vi "Fit Hall.vi"(11 "File Path":path=path "\\\\myhome\\NHMFL/Projects/Pressure/Code/Alex/m005_092123.tdms") -> ()   [LabVIEW 2023]
uses:
  <vilib>/Utility/file.llb/Write Delimited Spreadsheet (DBL).vi
  <vilib>/Analysis/NI_AALPro.lvlib
panel:
  in  "Save?":bool
  out "Waveform Graph":dbl[](graph)
  in  "X (Temperature)":dbl
  in  "file path (Fit results)":path
  out "Polynomial Coefficients":dbl[](array[numeric])
  in  "polynomial order":i32=2
  in  "Y":string="LakeShore 370 (18) R"
  in  "X":string="B"
  out "XY Graph":cluster{dbl[], dbl[]}[](graph)
  in  "group name in":string="p"
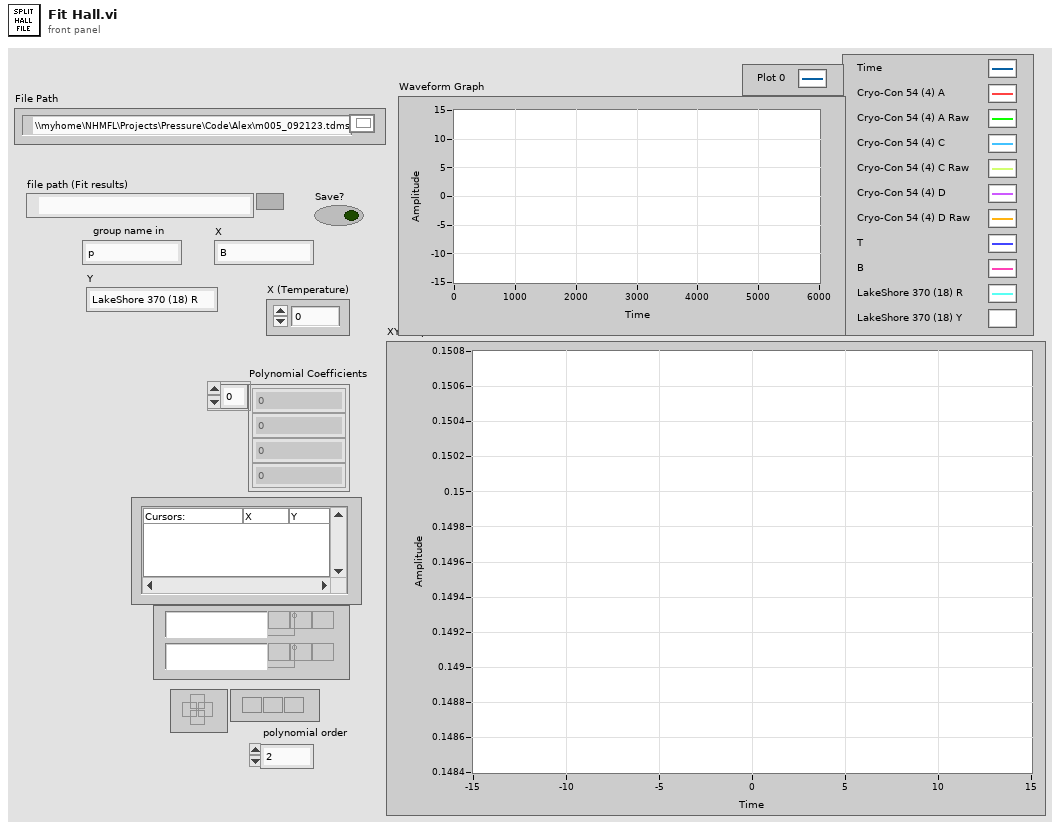
[diagram p1: front panel]
types:
  T1 = enum16{"open", "open or create", "create or replace", "create", "open (read-only)"}
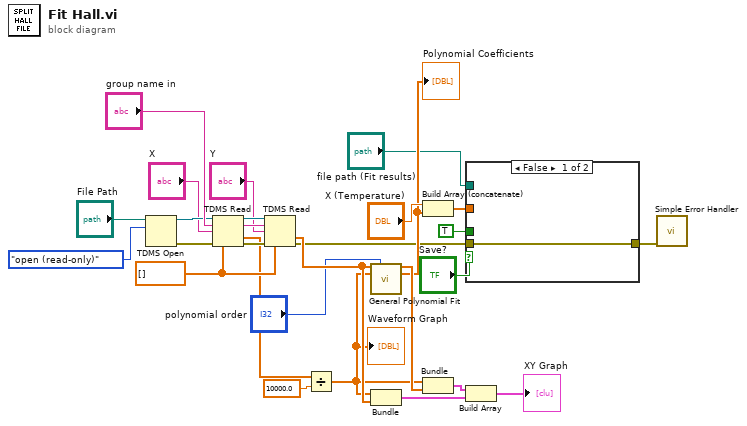
[diagram p0: block diagram]
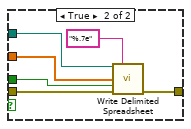
[diagram p2: hidden frame]
diagram:
  w20 = dbl[] []
  n1 = TDMS Open(10:T1."open (read-only)" ("operation (0:open)"), 11:"File Path") -> (0:w26:errorcluster, 3:w24:refnum<k34>)  [unwired: 5 in]
  n2 = TDMS Read(0:w24, 5:"group name in", 7:"X", 11:w26, 12:w20) -> (4:w23:refnum<k34>, 6:w21:string, 10:w11:dbl[], 15:w22:errorcluster)  [unwired: 3 in, 2 out]
  n3 = TDMS Read(0:w23, 5:w21, 7:"Y", 11:w22, 12:w20) -> (10:w17:dbl[], 15:w5:errorcluster)  [unwired: 3 in, 4 out]
  n4 = Divide(x=w11, y=10000.0) -> (x/y=w2:dbl[])
  "Waveform Graph" <- w2
  n5 = call <vilib>:"General Polynomial Fit.vi"("Y"=w17, "polynomial order"="polynomial order", "X"=w2) -> ("Best Polynomial Fit"=w15:dbl[], "Polynomial Coefficients"=w8:dbl[])  [unwired: 9 in, 2 out]
  "Polynomial Coefficients" <- w8
  n6 = Bundle(w2, w17) -> (w12:cluster{dbl[], dbl[]})  [unwired: 1 in]
  n7 = Build Array (concatenate)("X (Temperature)", w8) -> (w6:dbl[])
  n8 = Bundle(w2, "Best Polynomial Fit"=w15) -> (w13:cluster{dbl[], "Best Polynomial Fit":dbl[]})  [unwired: 1 in]
  n9 = case shown="False" "Save?" {
    tunnel: "file path (Fit results)" -> [_ w35]
    tunnel: w6 -> [_ w34]
    tunnel: w5 -> [w29 w33]
    tunnel: [w29 w32] -> w4
    tunnel: TRUE ("append to file? (new file:F)") -> [_ w31]
    frame False {
    }
    frame True {
      n10 = call-poly <vilib>:"Write Delimited Spreadsheet.vi"("file path (dialog if empty)"=w35, "format (%.3f)"="%.7e", "1D data"=w34, "append to file? (new file:F)"=w31, "error in (no error)"=w33) -> ("error out"=w32:errorcluster)  [unwired: 9 in, 1 out]
    }
  }
  n11 = Build Array(w13, w12) -> (→"XY Graph":cluster{dbl[], "Best Polynomial Fit":dbl[]}[])
  n12 = call <vilib>:"Simple Error Handler.vi"("error in (no error)"=w4) -> ()  [unwired: 4 in, 5 out]
